vi "Get New Transfer Identifier.vi"(8 "error in":errorcluster, 9 "label information":cluster{"label number":T1, "sdi":u8} {"label number" format="%.0o"}, 10 "channel number in":u8, 11 "board number in":u8) -> (0 "error out":errorcluster, 3 "Transfer ID out":u32, 5 "Transfer ID map":map{u32, u32}(c390))   [LabVIEW 2024, in "AIM ARINC 429 Hardware API.lvlib"]
uses:
  AIM ARINC 429 Hardware API.lvlib
  Shared/Label.ctl
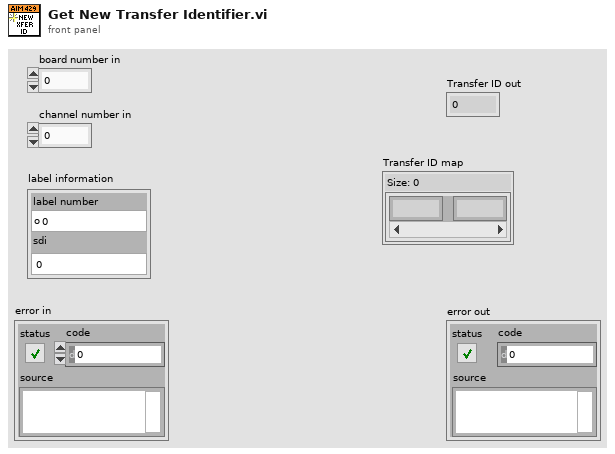
[diagram p1: front panel]
types:
  T1 = typedef "Label.ctl" = u8
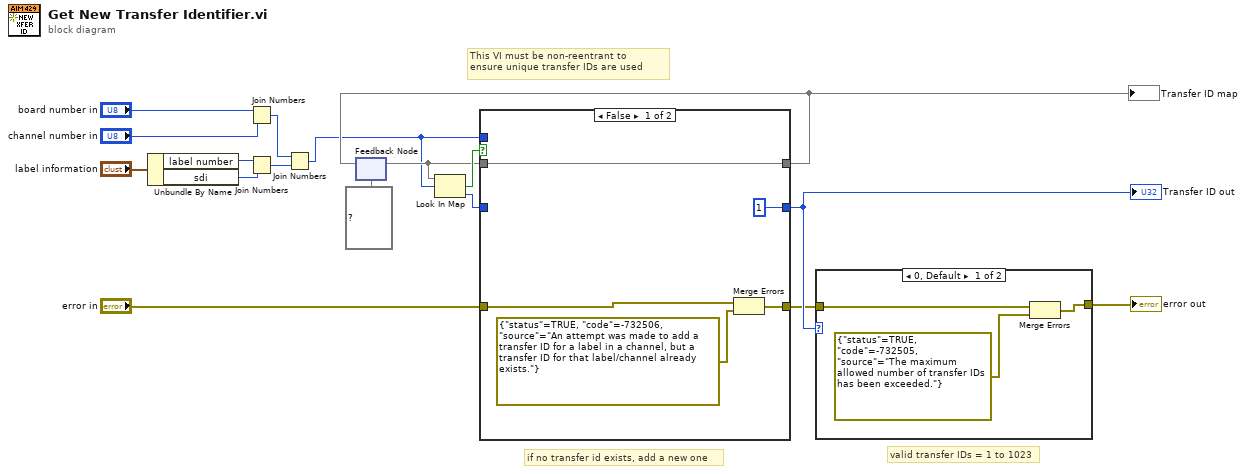
[diagram p0: block diagram]
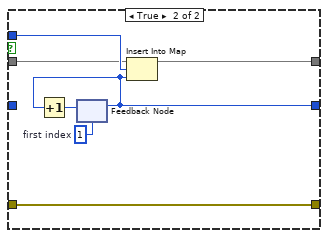
[diagram p2: hidden frame]
diagram:
  # "if no transfer id exists, add a new one"
  # "valid transfer IDs = 1 to 1023"
  # "This VI must be non-reentrant to \nensure unique transfer IDs are used"
  n1 = Unbundle By Name("label information") -> ("label number"=w7:T1, "sdi"=w6:u8)
  n2 = Join Numbers(hi="board number in", lo="channel number in") -> ((hi.lo)=w5:u16)
  n3 = Join Numbers(hi=w7, lo=w6) -> ((hi.lo)=w4:u16)
  n4 = Join Numbers(hi=w5, lo=w4) -> ((hi.lo)=w3:u32)
  n5 = feedback #1(map{u32, u32} {} ("map")) -> (w13:map{u32, u32})
  n6 = Look In Map(map=w13, key=w3) -> (key not found?=w15:bool, value=w14:u32)  [unwired: 1 in]
  n7 = case shown="False" w15 {
    tunnel: [u32 1 ("first index") w24] -> w11
    tunnel: w14 -> [_ _]
    tunnel: w13 -> [w22 w26]
    tunnel: w3 -> [_ w27]
    tunnel: [w22 w25] -> w12
    tunnel: [w20 w23] -> w2
    tunnel: "error in" -> [w19 w23]
    frame False {
      n8 = Merge Errors(w19, errorcluster {"status"=TRUE, "code"=-732506, "source"="An attempt was made to add a transfer ID for a label in a channel, but a transfer ID for that label/channel already exists."} ("error constant")) -> (w20:errorcluster)
    }
    frame True {
      w28 = u32 1  # first index
      n9 = feedback #2(w28) -> (w24:u32)
      n10 = Increment(x=w24) -> (x+1=w29:u32)
      n11 = feedback-in #2(w29) -> ()
      n12 = Insert Into Map(map in=w26, key=w27, value=w24) -> (map out=w25:map{u32, u32})  [unwired: 2 out]
    }
  }
  "Transfer ID out" <- w11
  "Transfer ID map" <- w12
  n13 = feedback-in #1(w12) -> ()
  n14 = case shown="0, Default" w11 {
    tunnel: [w32 w33] -> w17
    tunnel: w2 -> [w30 w33]
    frame 0, Default {
      n15 = Merge Errors(w30, errorcluster {"status"=TRUE, "code"=-732505, "source"="The maximum allowed number of transfer IDs has been exceeded."} ("error constant")) -> (w32:errorcluster)
    }
    frame 1..1023 {
    }
  }
  "error out" <- w17
